vi "Release CUDA dll (SubVI).vi"(1 "error in (no error)":errorcluster) -> (0 "error out":errorcluster)   [LabVIEW 2012]
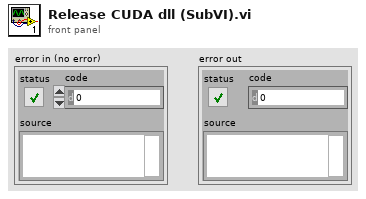
[diagram p1: front panel]
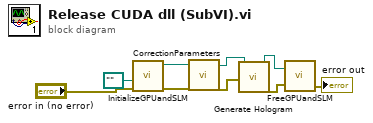
[diagram p0: block diagram]
diagram:
  n1 = call "InitializeGPUandSLM.vi"("CUDA/SLM error in (no error)"="error in (no error)", "dll path"=path "") -> ("CUDA/SLM error"=w5:errorcluster, "path out"=w2:path)  [unwired: 3 in, 1 out]
  n2 = call "CorrectionParameters.vi"("path in"=w2, "error in"=w5) -> ("path out"=w3:path, "error out"=w6:errorcluster)  [unwired: 23 in, 1 out]
  n3 = call "Generate Hologram.vi"("CUDA/SLM error in"=w6, "path in"=w3) -> ("path out"=w4:path, "CUDA/SLM error out"=w7:errorcluster)  [unwired: 21 in, 3 out]
  n4 = call "FreeGPUandSLM.vi"("path in"=w4, "error in"=w7) -> ("error out"=→"error out":errorcluster)  [unwired: 2 out]
